vi "Record_frame.vi"(8 "Ch in":cluster{i32, i32, i32, i32}={50, 650, 450, 1024}, 9 "Image Dst":T2, 10 "Image Src":T2, 11 "AVI Refnum in":T1) -> (2 "Image Out":T2, 3 "AVI Refnum out":T1)   [LabVIEW 2016]
uses:
  <vilib>/vision/Image Controls.llb/IMAQ Image.ctl
  <vilib>/vision/Avi.llb/IMAQ AVI2 Refnum.ctl
  <vilib>/vision/NI_Vision_Development_Module.lvlib
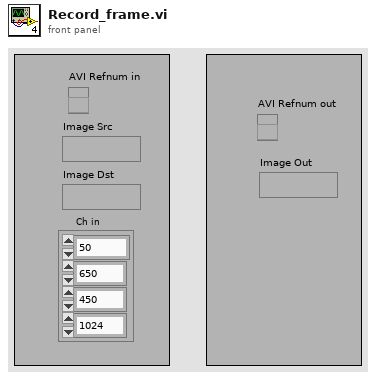
[diagram p1: front panel]
types:
  T1 = typedef "IMAQ AVI2 Refnum.ctl" = refnum<k20>
  T2 = typedef "IMAQ Image.ctl" = refnum<image>
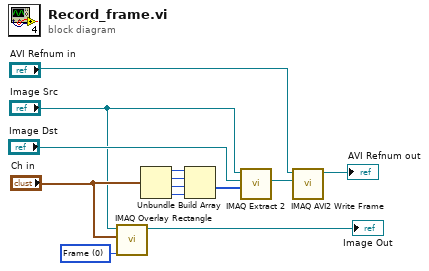
[diagram p0: block diagram]
diagram:
  w6 = u32 0 items=["Frame", "Fill", "Highlight"] ("Drawing Mode (Frame)")
  n1 = call "IMAQ Overlay Rectangle"("Drawing Mode (Frame)"=w6, "Rectangle"="Ch in", "Image"="Image Src") -> ("Image Out"=→"Image Out":T2)  [unwired: 7 in, 1 out]
  n2 = Unbundle("Ch in") -> (w10:i32, w9:i32, w8:i32, w7:i32)
  n3 = Build Array(w10, w9, w8, w7) -> (w11:i32[])
  n4 = call "IMAQ Extract 2"("Optional Rectangle"=w11, "Image Dst"="Image Dst", "Image Src"="Image Src") -> ("Image Dst Out"=w13:T2)  [unwired: 7 in, 1 out]
  n5 = call "IMAQ AVI2 Write Frame"("Image"=w13, "AVI Refnum"="AVI Refnum in") -> ("AVI Refnum (duplicate)"=→"AVI Refnum out":T1)  [unwired: 7 in, 2 out]
